vi "Check mtcdt check bt scan.vi"(6 "VISA resource name":refnum<visa-resource-name>="COM5", 7 "Passed so far":bool, 8 "error in (no error)":errorcluster) -> (0 "error out":errorcluster, 3 "BT mac":string, 4 "VISA Refnum out":refnum<visa-resource-name>, 5 "Passed?":bool)   [LabVIEW 2024]
panel:
  out "Response 5":string
  out "Response 2":string
  out "Response":string
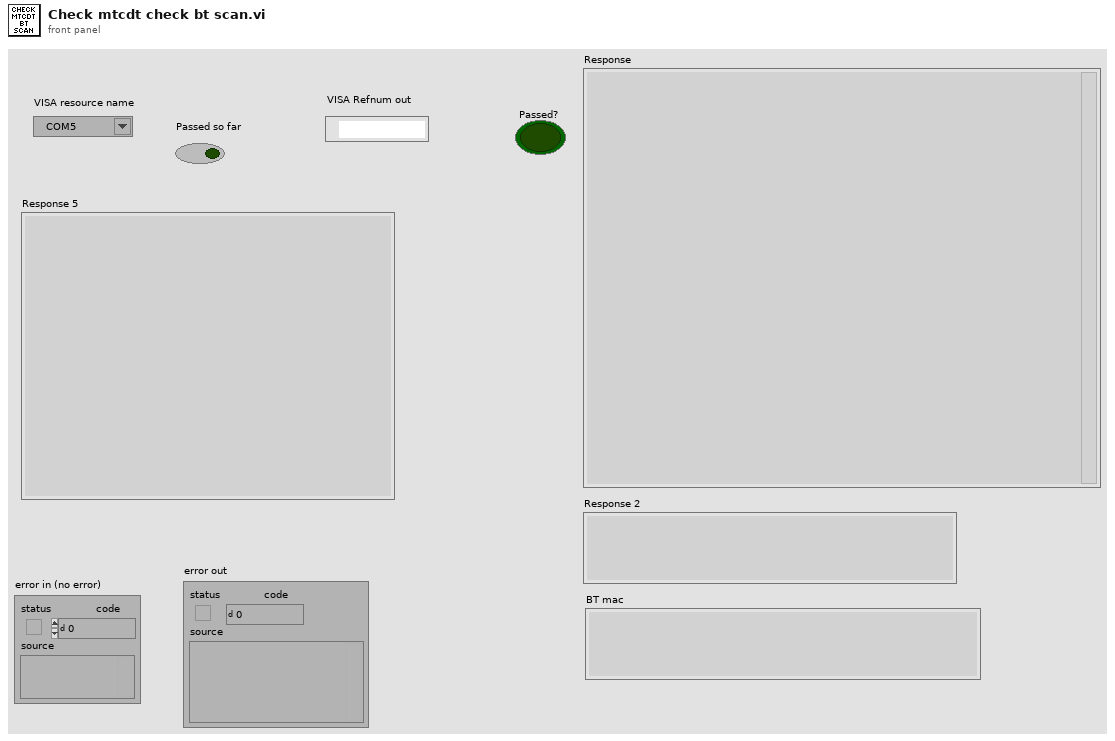
[diagram p1: front panel]
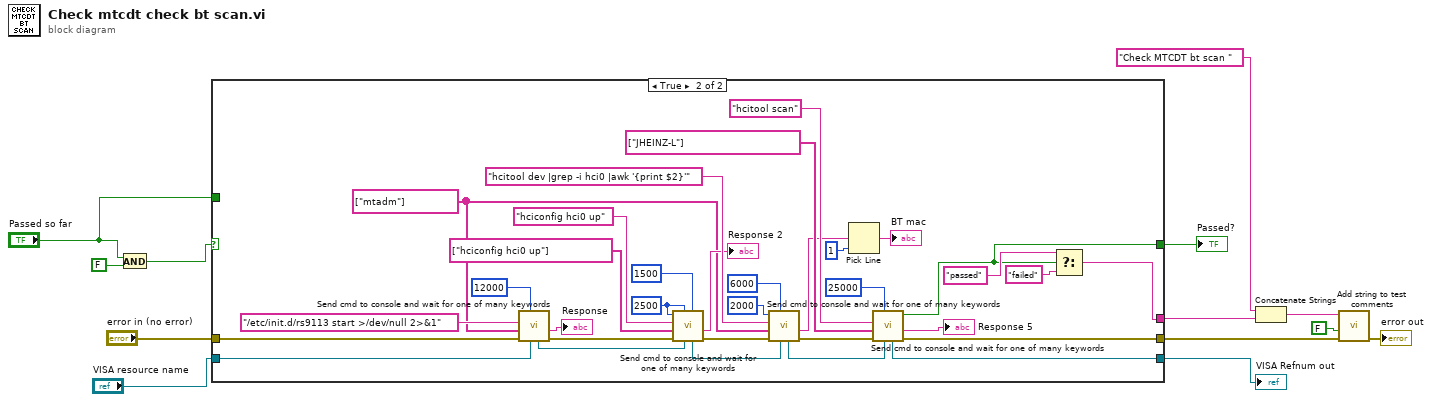
[diagram p0: block diagram]
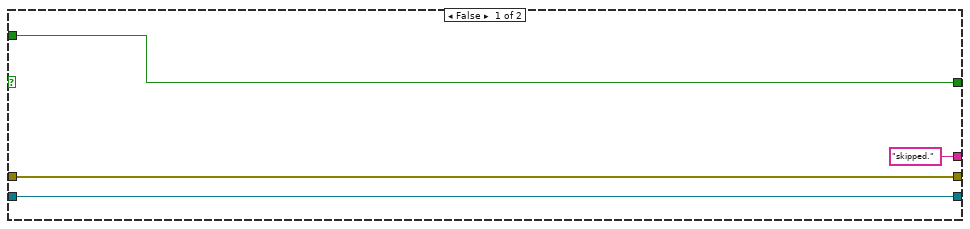
[diagram p2: hidden frame]
diagram:
  n1 = And(x="Passed so far", y=FALSE) -> (x .and. y?=w2:bool)
  n2 = case shown="True" w2 {
    tunnel: "error in (no error)" -> [w17 w37]
    tunnel: [w17 w32] -> w4
    tunnel: "VISA resource name" -> [w16 w29]
    tunnel: [w14 w31] -> w9
    tunnel: [w16 w30] -> w7
    tunnel: ["skipped." w34] -> w8
    tunnel: "Passed so far" -> [w14 _]
    frame False {
    }
    frame True {
      w24 = u32 2500 ("Wait after send")
      w26 = string[] ["mtadm"] ("Wait for keywords")
      n3 = call "Send cmd to console and wait for one of many keywords.vi"("VISA resource name"=w29, "Timeout (1000 mSecs)"=u32 12000, "error in (no error)"=w37, "Wait for keywords"=w26, "cmd"="/etc/init.d/rs9113 start >/dev/null 2>&1") -> ("error out"=w47:errorcluster, "Response"=→"Response":string, "VISA Refnum out"=w49:refnum<visa-resource-name>)  [unwired: 2 in, 2 out]
      n4 = call "Send cmd to console and wait for one of many keywords.vi"("Wait msecs after cmd ends (500ms)"=u32 1500, "VISA resource name"=w49, "Timeout (1000 mSecs)"=w24, "error in (no error)"=w47, "Wait for keywords"=string[] ["hciconfig hci0 up"], "cmd"="hciconfig hci0 up" ("write buffer"), "Wait after send"=w24) -> ("error out"=w45:errorcluster, "Response"=→"Response 2":string, "VISA Refnum out"=w44:refnum<visa-resource-name>)  [unwired: 2 out]
      n5 = call "Send cmd to console and wait for one of many keywords.vi"("VISA resource name"=w44, "Timeout (1000 mSecs)"=u32 6000, "error in (no error)"=w45, "Wait for keywords"=w26, "cmd"="hcitool dev |grep -i hci0 |awk '{print $2}'" ("write buffer"), "Wait after send"=u32 2000) -> ("error out"=w28:errorcluster, "Response"=w21:string, "VISA Refnum out"=w27:refnum<visa-resource-name>)  [unwired: 1 in, 2 out]
      n6 = Pick Line(multi-line string=w21, line index=1) -> (output string=→"BT mac":string)  [unwired: 1 in]
      n7 = call "Send cmd to console and wait for one of many keywords.vi"("VISA resource name"=w27, "Timeout (1000 mSecs)"=u32 25000, "error in (no error)"=w28, "Wait for keywords"=string[] ["JHEINZ-L"], "cmd"="hcitool scan" ("write buffer")) -> ("error out"=w32:errorcluster, "Response"=→"Response 5":string, "Found key?"=w31:bool, "VISA Refnum out"=w30:refnum<visa-resource-name>)  [unwired: 2 in, 1 out]
      n8 = Select(t="passed", s=w31, f="failed") -> (s? t:f=w34:string)
    }
  }
  "Passed?" <- w9
  "VISA Refnum out" <- w7
  n9 = Concatenate Strings("Check MTCDT bt scan " ("string"), w8) -> (w12:string)
  n10 = call "Add string to test comments.vi"("error in (no error)"=w4, "New Section (y)?"=FALSE, "Comments"=w12) -> ("error out"=→"error out":errorcluster)  [unwired: 7 in, 1 out]
